vi "FRCts20_Backend_Test_Comment_PUT.vi"(7 "Request Index":u32, 8 "error in (no error)":errorcluster, 10 "Solution":bool=TRUE, 11 "Note Index":u32) -> (0 "error out":errorcluster, 1 "Time (ms)":u32, 2 "Status":string, 3 "Note Out":T1, 5 "Success":bool)   [LabVIEW 2014, in "FRCts20_Backend_TestCode.lvlib"]
uses:
  FRCts20_Backend_TestCode.lvlib
  FRCts20_Backend_API/FRCts20_Backend_API_Note.ctl
  FRCts20_Backend_API/FRCts20_Backend_API_Command_Note.ctl
  FRCts20_Backend_API/FRCts20_Backend_API_Comment.vi
  FRCts20_Backend_API/FRCts20_Backend_API.lvlib
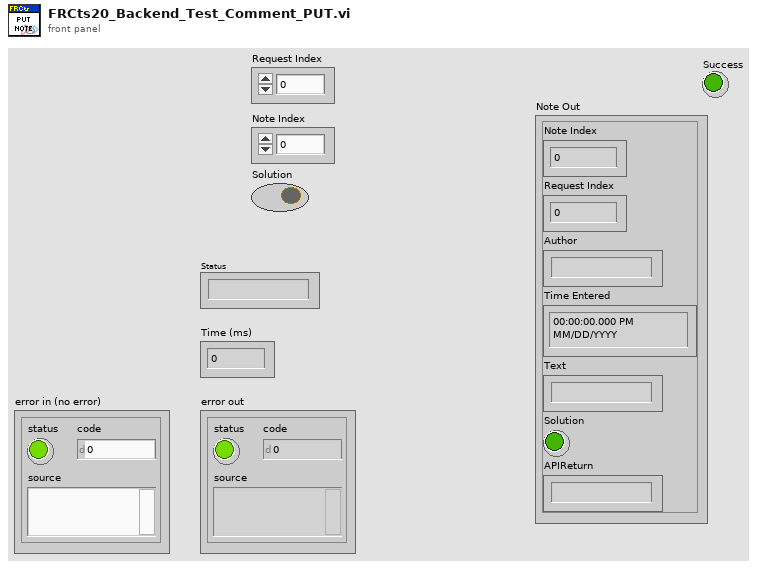
[diagram p1: front panel]
types:
  T1 = typedef "FRCts20_Backend_API.lvlib/FRCts20_Backend_API_Note.ctl" = cluster{"Note Index":u32, "Request Index":u32, "Author":string, "Time Entered":timestamp, "Text":string, "Solution":bool, "APIReturn":string}
  T2 = typedef "FRCts20_Backend_API.lvlib/FRCts20_Backend_API_Command_Note.ctl" = string
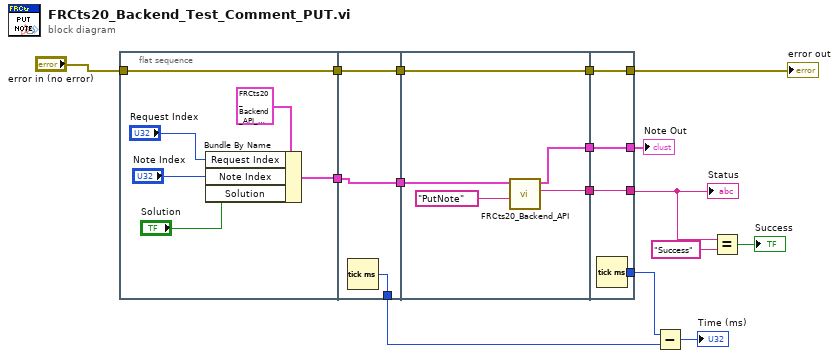
[diagram p0: block diagram]
diagram:
  n1 = flat-sequence {
    tunnel: [w22] -> w16
    tunnel: "error in (no error)" -> [w21]
    tunnel: [w21] -> w15
    tunnel: w16 -> [w23]
    tunnel: [w25] -> w8
    tunnel: [w24] -> w14
    tunnel: w15 -> [w24]
    tunnel: [w23] -> w2
    tunnel: [w30] -> w13
    tunnel: [w29] -> w12
    tunnel: [w28] -> w11
    tunnel: w14 -> [w28]
    tunnel: w2 -> [w26]
    tunnel: w13 -> [w34]
    tunnel: w12 -> [w33]
    tunnel: [w34] -> w5
    tunnel: [w33] -> w1
    tunnel: [w32] -> w7
    tunnel: [w31] -> w10
    tunnel: w11 -> [w31]
    frame #0 {
      n2 = Bundle By Name(cluster=T1 {"Note Index"=0, "Request Index"=0, "Author"="", "Time Entered"=timestamp(0 s since 1904-01-01), "Text"="", "Solution"=FALSE, "APIReturn"=""} ("Note In"), "Request Index"="Request Index", "Note Index"="Note Index", "Solution"="Solution") -> (w22:T1)
    }
    frame #1 {
      n3 = Tick Count (ms)() -> (millisecond timer value=w25:u32)
    }
    frame #2 {
      n4 = call-poly "FRCts20_Backend_API.vi"("Command"=T2 "PutNote", "Note In"=w26) -> ("Status"=w30:string, "Note Out"=w29:T1)  [unwired: 7 in, 1 out]
    }
    frame #3 {
      n5 = Tick Count (ms)() -> (millisecond timer value=w32:u32)
    }
  }
  n6 = Subtract(x=w7, y=w8) -> (x-y=→"Time (ms)":u32)
  n7 = Equal?(x=w5, y="Success") -> (x = y?=→"Success":bool)
  "error out" <- w10
  "Status" <- w5
  "Note Out" <- w1
